vi "Begin.vi"(8 "error in":errorcluster) -> (0 "error out":errorcluster)   [LabVIEW 2018]
doc: "Called before other user functions, this VI is expected to open initial I/O refnums, load in file data, and do all program initialization. Notice that the <B>error out</B> terminal is simply used for data flow. Wiring it to other structures or subVIs ensures that this VI runs first."
uses:
  <vilib>/Rock Robotics/WPI/DriverStation/WPI_DriverStationRobotMode2.ctl
  <vilib>/Rock Robotics/SystemInterfaces/AI/FPGA_AIChannel.ctl
  <vilib>/Rock Robotics/SystemInterfaces/DIO/FPGA_DIOPWMChannel.ctl
  <vilib>/Rock Robotics/SystemInterfaces/DIO/FPGA_DIOChannel.ctl
  Robot Global Data.vi
  <vilib>/Rock Robotics/WPI/MotorControl/WPI_MotorControlOpen SPARK.vi
  <vilib>/Rock Robotics/WPI/Counter/WPI_CounterDigitalInputToDigitalSource.vi
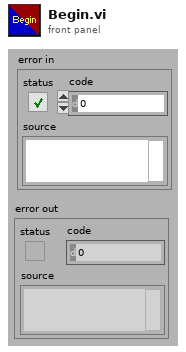
[diagram p1: front panel]
types:
  T1 = typedef "WPI_DriverStationRobotMode2.ctl" = enum16{"Autonomous Disabled", "Autonomous Enabled", "Teleop Disabled", "Teleop Enabled", "Disconnected", "Finish", "Test Disabled", "Test Enabled", "Emergency Stopped"}
  T2 = typedef "FPGA_AIChannel.ctl" = enum8{"AI 0", "AI 1", "AI 2", "AI 3", "AI MXP 0", "AI MXP 1", "AI MXP 2", "AI MXP 3", "Invalid"}
  T3 = typedef "FPGA_DIOPWMChannel.ctl" = enum8{"PWM 0", "PWM 1", "PWM 2", "PWM 3", "PWM 4", "PWM 5", "PWM 6", "PWM 7", "PWM 8", "PWM 9", "PWM MXP 0", "PWM MXP 1", "PWM MXP 2", "PWM MXP 3", "PWM MXP 4", "PWM MXP 5", "PWM MXP 6", "PWM MXP 7", "PWM MXP 8", "PWM MXP 9", "Invalid"}
  T4 = typedef "WPI_MotorControlDeviceRef.ctl" = cluster{"DeviceStatus":errorcluster, "Type":T5, "PWM":cluster{"PWM Channel":T3, "DeadBand":T6}, "CAN":cluster{"Device Number":u8, "SetOutput VI Ref":variant, "GetOutput VI Ref":variant, "Enable VI Ref":variant, "Disable VI Ref":variant, "Data":variant}, "Invert":bool, "DIO PWM":cluster{"PWM \"Enable\" Channel":T3, "DIOChannel":T7, "PWM Rate":dbl}}
  T5 = typedef "WPI_MotorControlType.ctl" = enum16{"PWM", "CAN", "DIO PWM"}
  T6 = typedef "WPI_PWMDeadband.ctl" = cluster{"Name":string, "maxPositivePwm":i32, "minPositivePwm":i32, "centerPwm":i32, "maxNegativePwm":i32, "minNegativePwm":i32, "angularRange":u16}
  T7 = typedef "FPGA_DIOChannel.ctl" = enum8{"DIO 0", "DIO 1", "DIO 2", "DIO 3", "DIO 4", "DIO 5", "DIO 6", "DIO 7", "DIO 8", "DIO 9", "DIO MXP 0", "DIO MXP 1", "DIO MXP 2", "DIO MXP 3", "DIO MXP 4", "DIO MXP 5", "DIO MXP 6", "DIO MXP 7", "DIO MXP 8", "DIO MXP 9", "DIO MXP 10", "DIO MXP 11", "DIO MXP 12", "DIO MXP 13", "DIO MXP 14", "DIO MXP 15", "SPI Port CS1", "SPI Port CS2", "SPI Port CS3", "SPI Port MISO", "SPI Port MOSI", "Invalid"}
  T8 = typedef "WPI_AnalogChannelDevRef.ctl" = cluster{"DevStatus":errorcluster, "Analog Channel":T2}
  T9 = typedef "WPI_DigitalInputDevRef.ctl" = cluster{"DevStatus":errorcluster, "DIO Channel":T7}
  T10 = typedef "FPGA_CounterEncoderSourceConvertionLVSourceType.ctl" = cluster{"DevStatus":errorcluster, "AnalogTriggerMode?":bool, "DigitalMode":cluster{"DIO Channel":T11}, "AnalogTriggerMode":cluster{"AnalogTriggerIndex":T12, "OutputType":T13}}
  T11 = typedef "FPGA_DIODigitalSourceChannel.ctl" = enum8{"DIO 0", "DIO 1", "DIO 2", "DIO 3", "DIO 4", "DIO 5", "DIO 6", "DIO 7", "DIO 8", "DIO 9", "DIO MXP 0", "DIO MXP 1", "DIO MXP 2", "DIO MXP 3", "DIO MXP 4", "DIO MXP 5", "DIO MXP 6", "DIO MXP 7", "DIO MXP 8", "DIO MXP 9", "DIO MXP 10", "DIO MXP 11", "DIO MXP 12", "DIO MXP 13", "DIO MXP 14", "DIO MXP 15", "SPI Port CS1", "SPI Port CS2", "SPI Port CS3", "SPI Port MISO", "SPI Port MOSI", "Disabled"}
  T12 = typedef "FPGA_AnalogTriggerIndex.ctl" = enum8{"Trig 0", "Trig 1", "Trig 2", "Trig 3", "Trig 4", "Trig 5", "Trig 6", "Trig 7", "Invalid"}
  T13 = typedef "FPGA_AnalogTriggerOutType.ctl" = enum16{"InWindow", "TriggerState", "Rising", "Falling"}
  T14 = typedef "WPI_EncoderDevRef.ctl" = cluster{"DevStatus":errorcluster, "EncoderIndex":T15, "CounterIndex":T16, "DistancePerCount":dbl, "Decoding Type":T17}
  T15 = typedef "FPGA_EncoderIdx.ctl" = enum8{"Enc 0", "Enc 1", "Enc 2", "Enc 3", "Enc 4", "Enc 5", "Enc 6", "Enc 7", "Invalid"}
  T16 = typedef "FPGA_CounterCtrSystemIndex.ctl" = enum8{"Ctr 0", "Ctr 1", "Ctr 2", "Ctr 3", "Ctr 4", "Ctr 5", "Ctr 6", "Ctr 7", "Invalid"}
  T17 = typedef "WPI_EncoderType.ctl" = enum16{"1x", "2x", "4x"}
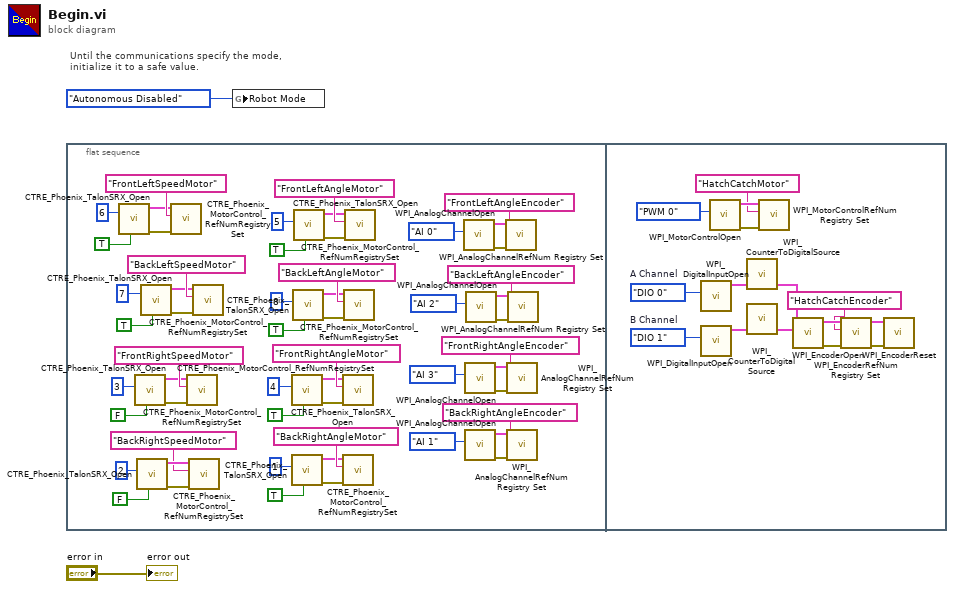
[diagram p0: block diagram]
diagram:
  # "Until the communications specify the mode,\ninitialize it to a safe value."
  n1 = flat-sequence {
    frame #0 {
      n2 = call <vilib>:"CTRE_Phoenix_TalonSRX_Open.vi"("Invert"=TRUE, "Device Number"=u8 6) -> ("error out"=w44:errorcluster, "CAN Talon SRX Ref"=w45:T4)  [unwired: 8 in]
      n3 = call <vilib>:"CTRE_Phoenix_TalonSRX_Open.vi"("Invert"=FALSE, "Device Number"=u8 3) -> ("error out"=w48:errorcluster, "CAN Talon SRX Ref"=w49:T4)  [unwired: 8 in]
      n4 = call <vilib>:"CTRE_Phoenix_TalonSRX_Open.vi"("Invert"=FALSE, "Device Number"=u8 2) -> ("error out"=w50:errorcluster, "CAN Talon SRX Ref"=w51:T4)  [unwired: 8 in]
      n5 = call <vilib>:"CTRE_Phoenix_TalonSRX_Open.vi"("Invert"=TRUE, "Device Number"=u8 7) -> ("error out"=w46:errorcluster, "CAN Talon SRX Ref"=w47:T4)  [unwired: 8 in]
      n6 = call <vilib>:"CTRE_Phoenix_MotorControl_RefNumRegistrySet.vi"("error in (no error)"=w44, "refnum name"="FrontLeftSpeedMotor", "PhoenixMotorControlDevRef"=w45) -> ()  [unwired: 7 in, 2 out]
      n7 = call <vilib>:"CTRE_Phoenix_MotorControl_RefNumRegistrySet.vi"("error in (no error)"=w48, "refnum name"="FrontRightSpeedMotor", "PhoenixMotorControlDevRef"=w49) -> ()  [unwired: 7 in, 2 out]
      n8 = call <vilib>:"CTRE_Phoenix_MotorControl_RefNumRegistrySet.vi"("error in (no error)"=w50, "refnum name"="BackRightSpeedMotor", "PhoenixMotorControlDevRef"=w51) -> ()  [unwired: 7 in, 2 out]
      n9 = call <vilib>:"CTRE_Phoenix_MotorControl_RefNumRegistrySet.vi"("error in (no error)"=w46, "refnum name"="BackLeftSpeedMotor", "PhoenixMotorControlDevRef"=w47) -> ()  [unwired: 7 in, 2 out]
      n10 = call <vilib>:"CTRE_Phoenix_TalonSRX_Open.vi"("Invert"=TRUE, "Device Number"=u8 4) -> ("error out"=w30:errorcluster, "CAN Talon SRX Ref"=w31:T4)  [unwired: 8 in]
      n11 = call <vilib>:"CTRE_Phoenix_TalonSRX_Open.vi"("Invert"=TRUE, "Device Number"=u8 1) -> ("error out"=w28:errorcluster, "CAN Talon SRX Ref"=w29:T4)  [unwired: 8 in]
      n12 = call <vilib>:"CTRE_Phoenix_TalonSRX_Open.vi"("Invert"=TRUE, "Device Number"=u8 8) -> ("error out"=w32:errorcluster, "CAN Talon SRX Ref"=w33:T4)  [unwired: 8 in]
      n13 = call <vilib>:"CTRE_Phoenix_TalonSRX_Open.vi"("Invert"=TRUE, "Device Number"=u8 5) -> ("error out"=w34:errorcluster, "CAN Talon SRX Ref"=w35:T4)  [unwired: 8 in]
      n14 = call <vilib>:"CTRE_Phoenix_MotorControl_RefNumRegistrySet.vi"("error in (no error)"=w30, "refnum name"="FrontRightAngleMotor", "PhoenixMotorControlDevRef"=w31) -> ()  [unwired: 7 in, 2 out]
      n15 = call <vilib>:"CTRE_Phoenix_MotorControl_RefNumRegistrySet.vi"("error in (no error)"=w28, "refnum name"="BackRightAngleMotor", "PhoenixMotorControlDevRef"=w29) -> ()  [unwired: 7 in, 2 out]
      n16 = call <vilib>:"CTRE_Phoenix_MotorControl_RefNumRegistrySet.vi"("error in (no error)"=w32, "refnum name"="BackLeftAngleMotor", "PhoenixMotorControlDevRef"=w33) -> ()  [unwired: 7 in, 2 out]
      n17 = call <vilib>:"CTRE_Phoenix_MotorControl_RefNumRegistrySet.vi"("error in (no error)"=w34, "refnum name"="FrontLeftAngleMotor", "PhoenixMotorControlDevRef"=w35) -> ()  [unwired: 7 in, 2 out]
      n18 = call <vilib>:"WPI_AnalogChannelOpen.vi"("Analog Channel"=FPGA_AIChannel."AI 0") -> ("error out"=w26:errorcluster, "AIDeviceRef"=w27:T8)  [unwired: 9 in]
      n19 = call <vilib>:"WPI_AnalogChannelOpen.vi"("Analog Channel"=FPGA_AIChannel."AI 3") -> ("error out"=w18:errorcluster, "AIDeviceRef"=w19:T8)  [unwired: 9 in]
      n20 = call <vilib>:"WPI_AnalogChannelOpen.vi"("Analog Channel"=FPGA_AIChannel."AI 1") -> ("error out"=w14:errorcluster, "AIDeviceRef"=w15:T8)  [unwired: 9 in]
      n21 = call <vilib>:"WPI_AnalogChannelOpen.vi"("Analog Channel"=FPGA_AIChannel."AI 2") -> ("error out"=w22:errorcluster, "AIDeviceRef"=w23:T8)  [unwired: 9 in]
      n22 = call <vilib>:"WPI_AnalogChannelRefNum Registry Set.vi"("error in (no error)"=w26, "refnum name"="FrontLeftAngleEncoder", "AIDeviceRef"=w27) -> ()  [unwired: 7 in, 2 out]
      n23 = call <vilib>:"WPI_AnalogChannelRefNum Registry Set.vi"("error in (no error)"=w18, "refnum name"="FrontRightAngleEncoder", "AIDeviceRef"=w19) -> ()  [unwired: 7 in, 2 out]
      n24 = call <vilib>:"WPI_AnalogChannelRefNum Registry Set.vi"("error in (no error)"=w14, "refnum name"="BackRightAngleEncoder", "AIDeviceRef"=w15) -> ()  [unwired: 7 in, 2 out]
      n25 = call <vilib>:"WPI_AnalogChannelRefNum Registry Set.vi"("error in (no error)"=w22, "refnum name"="BackLeftAngleEncoder", "AIDeviceRef"=w23) -> ()  [unwired: 7 in, 2 out]
    }
    frame #1 {
      w60 = FPGA_DIOChannel."DIO 1"  # B Channel
      w59 = FPGA_DIOChannel."DIO 0"  # A Channel
      n26 = call <vilib>:"WPI_DigitalInputOpen.vi"("DIO Channel"=w59) -> ("DigitalInputDevRef"=w64:T9)  [unwired: 1 in, 9 out]
      n27 = call <vilib>:"WPI_DigitalInputOpen.vi"("DIO Channel"=w60) -> ("DigitalInputDevRef"=w63:T9)  [unwired: 1 in, 9 out]
      n28 = call-poly <vilib>:"WPI_MotorControlOpen.vi"("PWM Channel"=FPGA_DIOPWMChannel."PWM 0") -> ("error out"=w73:errorcluster, "MotorControlDeviceRef"=w72:T4)  [unwired: 9 in]
      n29 = call-poly <vilib>:"WPI_CounterToDigitalSource.vi"("DigitalInputDevRef"=w64) -> ("Digital Source"=w65:T10)  [unwired: 6 out]
      n30 = call-poly <vilib>:"WPI_CounterToDigitalSource.vi"("DigitalInputDevRef"=w63) -> ("Digital Source"=w62:T10)  [unwired: 6 out]
      n31 = call <vilib>:"WPI_MotorControlRefNum Registry Set.vi"("error in (no error)"=w73, "refnum name"="HatchCatchMotor", "MotorControlDevRef"=w72) -> ()  [unwired: 7 in, 2 out]
      n32 = call <vilib>:"WPI_EncoderOpen.vi"("BSource"=w62, "ASource"=w65) -> ("error out"=w66:errorcluster, "EncoderDevRef"=w67:T14)  [unwired: 6 in, 2 out]
      n33 = call <vilib>:"WPI_EncoderRefNum Registry Set.vi"("error in (no error)"=w66, "refnum name"="HatchCatchEncoder", "EncoderDevRef"=w67) -> ("error out"=w68:errorcluster, "EncoderDevRef"=w69:T14)  [unwired: 7 in]
      n34 = call <vilib>:"WPI_EncoderReset.vi"("error in (no error)"=w68, "EncoderDevRef"=w69) -> ()  [unwired: 8 in, 2 out]
    }
  }
  n35 = global write "Robot Global Data.vi" "Robot Mode"(WPI_DriverStationRobotMode2."Autonomous Disabled" ("Robot Mode")) -> ()
  "error out" <- "error in"
